vi "Tokenize Command.vi"(8 "error in (no error)":errorcluster, 10 "switches in":string[](array[string]), 11 "command in":string) -> (0 "error out":errorcluster, 2 "switches out":cluster{"switch":string, "argument":string}[](array[cluster]), 3 "command out":string)   [LabVIEW 2017]
doc: "Parses <b>command in</b> and returns separated command with switches and switches arguments. Switch argument do not need to be surrounded by quotes.\n\nExample\ncommand in: cmd -a arg1 -b arg2\nswitches: -a, -b\ncommand out: cmd \nswitches out[0].switch: -a\nswitches out[0].argument: arg1\nswitches out[1].switch: -b\nswitches out[1].argument: arg2"
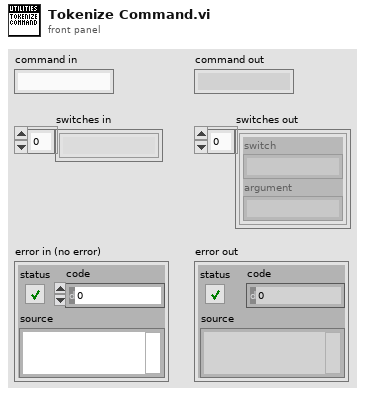
[diagram p1: front panel]
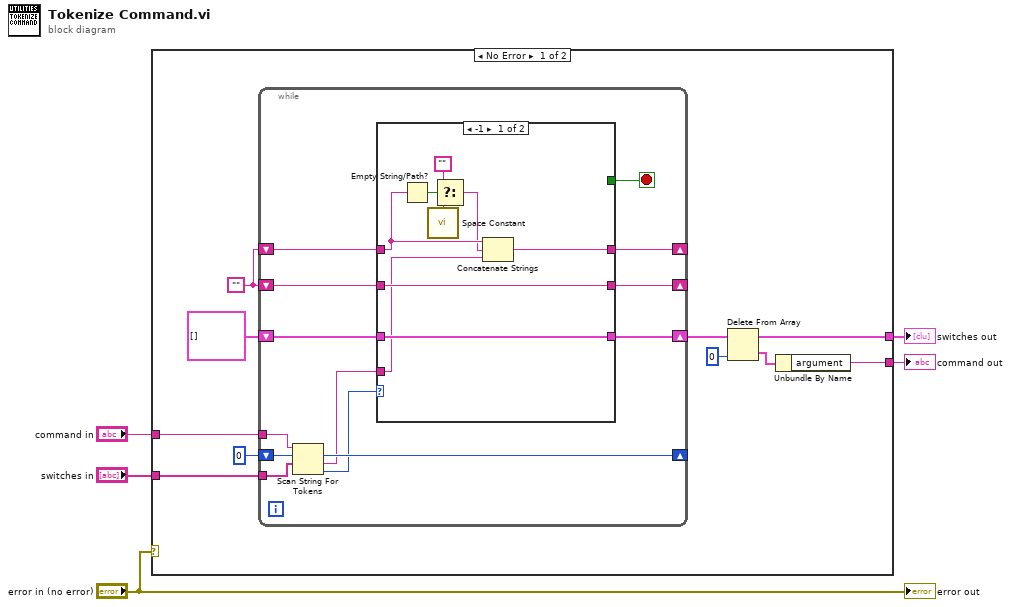
[diagram p0: block diagram]
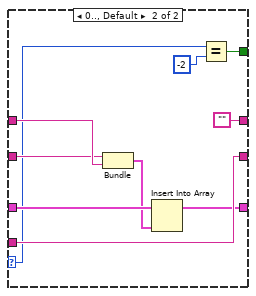
[diagram p2: hidden frame]
diagram:
  n1 = case shown="No Error" "error in (no error)" {
    tunnel: "switches in" -> [w12 _]
    tunnel: "command in" -> [w11 _]
    tunnel: [w9 _] -> w3
    tunnel: [w7 _] -> w2
    frame No Error {
      w14 = ""
      n2 = while {
        tunnel: w11 -> [w28]
        shift-right: [w27] -> _
        shift-left: 0 ("offset past token") -> [w26]
        tunnel: w12 -> [w25]
        shift-right: [w21] -> _
        shift-left: w14 -> [w18]
        shift-right: [w20] -> _
        shift-left: w14 -> [w19]
        shift-right: [w17] -> w10
        shift-left: cluster{"switch":string, "argument":string}[] [] -> [w16]
        stop <- w23 stop-if-true
        n3 = Scan String For Tokens(7:w25, 8:w26, 9:w28) -> (0:w24:i32, 1:w22:string, 2:w27:i32)  [unwired: 3 in, 1 out]
        n4 = case shown="-1" w24 {
          selector: w24 -> [_ w40]
          tunnel: [_ w38] -> w23
          tunnel: w22 -> [w34 w45]
          tunnel: [w36 w45] -> w21
          tunnel: [w37 ""] -> w20
          tunnel: w19 -> [w33 w44]
          tunnel: w18 -> [w36 w41]
          tunnel: [w35 w42] -> w17
          tunnel: w16 -> [w35 w47]
          frame -1 {
            n5 = Empty String/Path?(string/path=w33) -> (empty?=w32:bool)
            n6 = call <vilib>:"Space Constant.vi"() -> ("String"=w30:string)
            n7 = Select(t="", s=w32, f=w30) -> (s? t:f=w29:string)
            n8 = Concatenate Strings(w33, w29, w34) -> (w37:string)
          }
          frame 0.., Default {
            n9 = Bundle(w41, w44) -> (w43:cluster{string, string})  [unwired: 1 in]
            n10 = Insert Into Array(array=w47, new element=w43) -> (w42:cluster{"switch":string, "argument":string}[])  [unwired: 1 in]
            n11 = Equal?(x=w40, y=-2) -> (x = y?=w38:bool)
          }
        }
      }
      n12 = Delete From Array(array=w10, index=0) -> (deleted portion=w8:cluster{"switch":string, "argument":string}, array with subset deleted=w9:cluster{"switch":string, "argument":string}[])  [unwired: 1 in]
      n13 = Unbundle By Name(w8) -> ("argument"=w7:string)
    }
    frame Error {
    }
  }
  "switches out" <- w3
  "command out" <- w2
  "error out" <- "error in (no error)"
